vi "p42 mascara puntos de interes.vi"() -> ()   [LabVIEW 2017]
panel:
  out "new picture 2":picture
  in  "Slide":dbl(slide) scale=0.0..255.0
  in  "path to BMP file":path
  out "new picture":picture
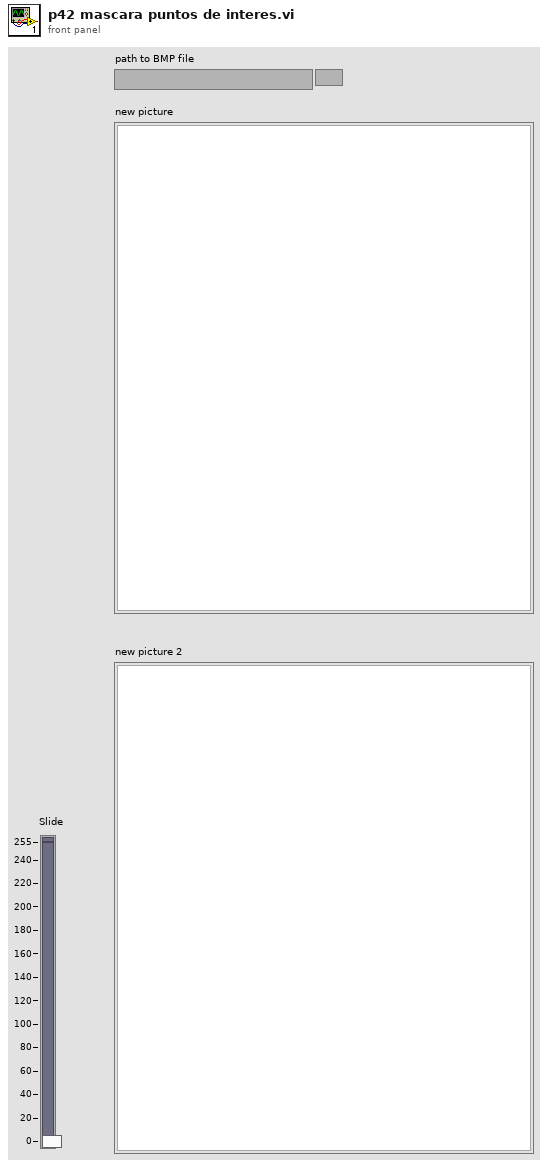
[diagram p1: front panel]
types:
  T1 = typedef "imagedata.ctl" = cluster{"image type":i32, "image depth":i32, "image":u8[], "mask":u8[], "colors":u32[], "Rectangle":cluster{"left":i16, "top":i16, "right":i16, "bottom":i16}}
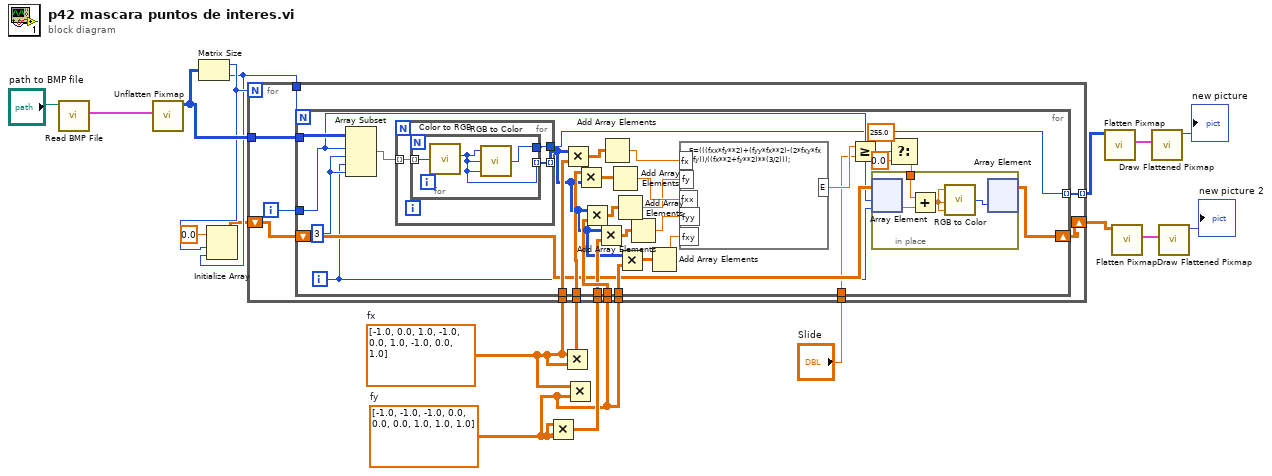
[diagram p0: block diagram]
diagram:
  w10 = dbl[][] [[-1.0, -1.0, -1.0], [0.0, 0.0, 0.0], [1.0, 1.0, 1.0]]  # fy
  w13 = dbl[][] [[-1.0, 0.0, 1.0], [-1.0, 0.0, 1.0], [-1.0, 0.0, 1.0]]  # fx
  n1 = call <vilib>:"Read BMP File.vi"("path to BMP file"="path to BMP file") -> ("image data"=w15:T1)  [unwired: 8 in, 2 out]
  n2 = call <vilib>:"Unflatten Pixmap.vi"("image data"=w15) -> ("24-bit pixmap"=w14:u32[][])  [unwired: 4 in, 6 out]
  n3 = Matrix Size(0:w14) -> (1:w8:i32, 2:w7:i32)
  n4 = Initialize Array(0.0 ("element"), w8, w7) -> (w6:dbl[][])
  n5 = Multiply(x=w10, y=w10) -> (x*y=w11:dbl[][])
  n6 = Multiply(x=w13, y=w13) -> (x*y=w12:dbl[][])
  n7 = for {
    N: w8 -> [_]
    tunnel: w14 -> [w30]
    tunnel: w7 -> [w28]
    tunnel: w13 -> [w27]
    tunnel: w12 -> [w26]
    tunnel: w10 -> [w25]
    tunnel: w11 -> [w24]
    tunnel: w10 -> [w23]
    tunnel: [w21] -> w5 mode=indexing
    tunnel: "Slide" -> [w20]
    shift-right: [w19] -> w1
    shift-left: w6 -> [w22]
    i -> [w29]
    n8 = for {
      N: w28 -> [_]
      tunnel: w30 -> [w60]
      tunnel: w29 -> [w40]
      tunnel: w27 -> [w57]
      tunnel: w26 -> [w56]
      tunnel: w25 -> [w55]
      tunnel: w24 -> [w54]
      tunnel: w23 -> [w44]
      tunnel: [w38] -> w21 mode=indexing
      tunnel: w20 -> [w35]
      shift-right: [w31] -> w19
      shift-left: w22 -> [w41]
      i -> [w39]
      w59 = 3
      n9 = Array Subset(array=w60, index (row)=w40, length (row)=w59, index (col)=w39, length (col)=w59) -> (w58:u32[][])
      n10 = for {
        tunnel: w58 -> [w67] mode=indexing
        tunnel: [w66] -> w45 mode=indexing
        tunnel: [w65] -> w38
        n11 = for {
          tunnel: w67 -> [w70] mode=indexing
          tunnel: [w69] -> w66 mode=indexing
          tunnel: [w68] -> w65
          n12 = call <vilib>:"Color to RGB.vi"("Color"=w70) -> ("R"=w69:u8)  [unwired: 3 out]
          n13 = call <vilib>:"RGB to Color.vi"("B"=w69, "G"=w69, "R"=w69) -> ("Color"=w68:u32)
        }
      }
      n14 = Multiply(x=w45, y=w57) -> (x*y=w53:dbl[][])
      n15 = Multiply(x=w56, y=w45) -> (x*y=w51:dbl[][])
      n16 = Multiply(x=w45, y=w55) -> (x*y=w49:dbl[][])
      n17 = Multiply(x=w45, y=w54) -> (x*y=w47:dbl[][])
      n18 = Add Array Elements(numeric array=w53) -> (sum=w52:dbl)
      n19 = Add Array Elements(numeric array=w51) -> (sum=w50:dbl)
      n20 = Add Array Elements(numeric array=w49) -> (sum=w48:dbl)
      n21 = Multiply(x=w45, y=w44) -> (x*y=w42:dbl[][])
      n22 = Add Array Elements(numeric array=w47) -> (sum=w46:dbl)
      n23 = Add Array Elements(numeric array=w42) -> (sum=w43:dbl)
      n24 = formula code="E=(((fxx*fy**2)+(fyy*fx**2)-(2*fxy*fx*fy))/((fx**2+fy**2)**(3/2)));"("fx"=w52, "fy"=w48, "fxx"=w50, "fyy"=w46, "fxy"=w43) -> ("E"=w36:dbl)
      n25 = Greater Or Equal?(x=w36, y=w35) -> (x >= y?=w37:bool)
      n26 = Select(t=255.0, s=w37, f=0.0) -> (s? t:f=w32:dbl)
      n27 = in-place {
        in-place-border: w32 -> [w63]
        n28 = in-place-array #1(w41, w40, w39) -> (w64:dbl)
        n29 = Add(x=w63, y=w64) -> (x+y=w62:dbl)
        n30 = call <vilib>:"RGB to Color.vi"("B"=w62, "G"=w62, "R"=w62) -> ("Color"=w61:u32)
        n31 = in-place-array #1(w61) -> (w31:dbl[][])  [unwired: 2 out]
      }
    }
  }
  n32 = Multiply(x=w13, y=w10) -> ()  [unwired: 1 out]
  n33 = call <vilib>:"Flatten Pixmap.vi"("24-bit pixmap"=w5) -> ("image data"=w18:T1)  [unwired: 10 in]
  n34 = call <vilib>:"Flatten Pixmap.vi"("24-bit pixmap"=w1) -> ("image data"=w2:T1)  [unwired: 10 in]
  n35 = call <vilib>:"Draw Flattened Pixmap.vi"("image data"=w18) -> ("new picture"=→"new picture":picture)  [unwired: 8 in]
  n36 = call <vilib>:"Draw Flattened Pixmap.vi"("image data"=w2) -> ("new picture"=→"new picture 2":picture)  [unwired: 8 in]
